vi "Set Trigger.vi"(8 "error in (no error)":errorcluster, 10 "Trigger Settings":T1={"Edge:"=0, "Level"=0.0, "Source"=0, "trigger coupling"=1, "Holdoff"=0.0, "Delay"=0.0, "Trigger Modifier"=enum."Auto Trigger", "Trigger Type"=enum."Digital"} {"trigger coupling" items=["AC", "DC", "HF Reject", "LF Reject", "AC Plus HF Reject"]; "Source" items=["Channel_1", "Channel_2", "Channel_3", "Channel_4", "Channel_5", "Channel_6", "Channel_7", "Channel_8"]; "Edge:" items=["Rising Edge", "Falling Edge"]}, 11 "Oscilloscope in":refnum<class "Oscilloscope.lvclass">) -> (0 "error out":errorcluster, 3 "Oscilloscope out":refnum<class "Oscilloscope.lvclass">)   [LabVIEW 2019, in "Oscilloscope.lvlib" / "Oscilloscope.lvclass"]
uses:
  Oscilloscope.lvclass
  Custom Controls/Trigger Settings.ctl
  Custom Controls/Edge Select.ctl
  Custom Controls/Channel List.ctl
  Custom Controls/Trigger Coupling.ctl
  Custom Controls/Trigger Modifier.ctl
  Custom Controls/Trigger Type.ctl
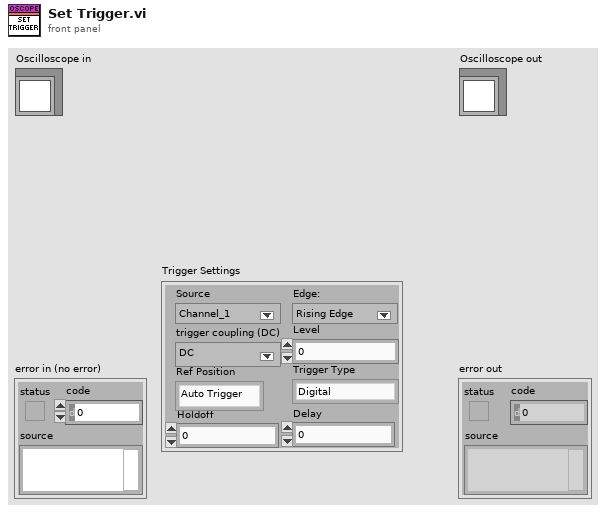
[diagram p1: front panel]
types:
  T1 = typedef "Oscilloscope.lvlib/Oscilloscope.lvclass/Trigger Settings.ctl" = cluster{"Edge:":T2, "Level":dbl, "Source":T3, "trigger coupling":T4, "Holdoff":dbl, "Delay":dbl, "Trigger Modifier":T5, "Trigger Type":T6}
  T2 = typedef "Oscilloscope.lvlib/Oscilloscope.lvclass/Edge Select.ctl" = u16
  T3 = typedef "Oscilloscope.lvlib/Oscilloscope.lvclass/Channel List.ctl" = u16
  T4 = typedef "Oscilloscope.lvlib/Oscilloscope.lvclass/Trigger Coupling.ctl" = u16
  T5 = typedef "Oscilloscope.lvlib/Oscilloscope.lvclass/Trigger Modifier.ctl" = enum16{"Invalid_Setting", "None", "Auto Trigger"}
  T6 = typedef "Oscilloscope.lvlib/Oscilloscope.lvclass/Trigger Type.ctl" = enum16{"Immediate", "Analog Edge", "Digital", "Window", "Hysteresis"}
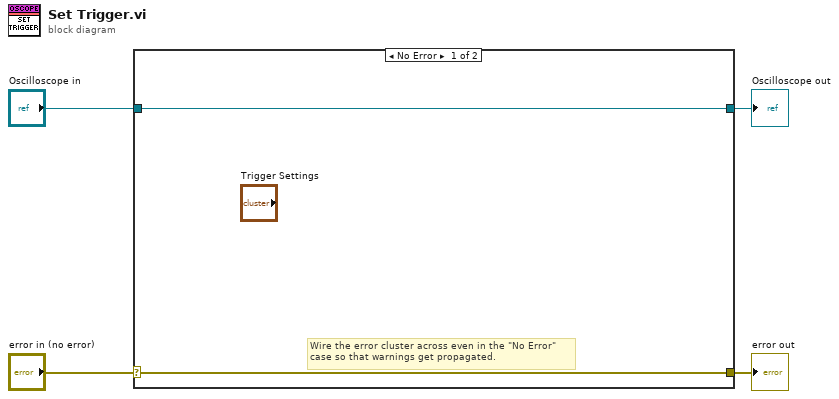
[diagram p0: block diagram]
diagram:
  n1 = case shown="No Error" "error in (no error)" {
    selector: "error in (no error)" -> [w5 w8]
    tunnel: [w5 w8] -> w3
    tunnel: [w6 w7] -> w1
    tunnel: "Oscilloscope in" -> [w6 w7]
    frame No Error {
      # "Wire the error cluster across even in the \"No Error\"\ncase so that warnings get propagated."
    }
    frame Error {
    }
  }
  "error out" <- w3
  "Oscilloscope out" <- w1
